vi "Select All Positions for Curve Fit.vi"(1 "Max Positions per Rack":i32, 2 "Rack Status In":bool[](array[boolean]), 3 "Active Positions":bool[](array[boolean])) -> (0 "Rack Status Out":bool[](array[boolean]))   [LabVIEW 2021]
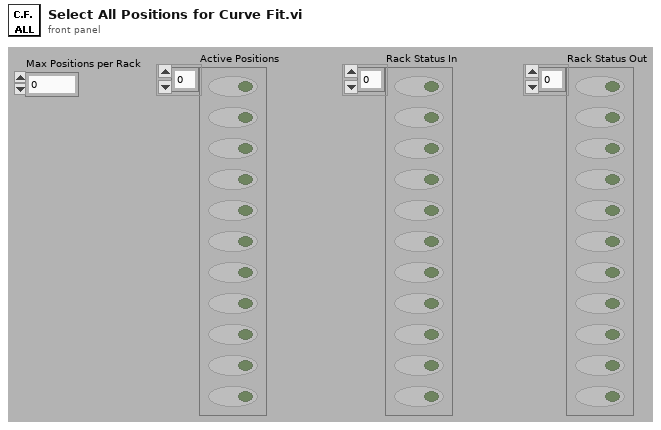
[diagram p1: front panel]
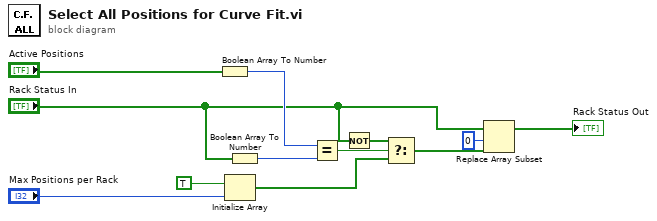
[diagram p0: block diagram]
diagram:
  n1 = Boolean Array To Number(Boolean array="Active Positions") -> (number=w10:u32)
  n2 = Initialize Array(TRUE, "Max Positions per Rack") -> (w3:bool[])
  n3 = Boolean Array To Number(Boolean array="Rack Status In") -> (number=w8:u32)
  n4 = Equal?(x=w10, y=w8) -> (x = y?=w11:bool)
  n5 = Not(x="Rack Status In") -> (.not. x?=w5:bool[])
  n6 = Select(t=w5, s=w11, f=w3) -> (s? t:f=w7:bool[])
  n7 = Replace Array Subset(array="Rack Status In", new element=w7, index=0) -> (→"Rack Status Out":bool[])
